vi "Sans titre 2.vi"() -> ()   [LabVIEW 2010]
uses:
  \\iutehc-filer\ourion5/PortableGit-2.11.0.3-64-bit.7z/actniet/act/lv_01/lv_01.lvlib
panel:
  in  "x":dbl[](array[numeric])
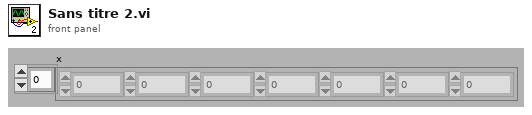
[diagram p1: front panel]
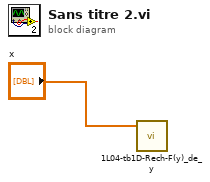
[diagram p0: block diagram]
diagram:
  n1 = call "1L04-tb1D-Rech-F(y)_de_y.vi"("x"="x") -> ()  [unwired: 2 in, 1 out]
